vi "sub2.vi"(10 "regular expression":string, 11 "Array":T1(array[cluster])) -> (3 "Tunnel out":refnum<vi>)   [LabVIEW 2020, in "CSM-Helper.lvclass"]
uses:
  CSM-Helper.lvclass
  a22f351f-3913-4f37-956c-d0ef2cfe06c6.vi
  cf7c94ff-430a-4fdd-9615-a1dbd9b9f88c.vi
  a22f351f-3913-4f37-956c-d0ef2cfe06c6.vi/eb2405bd-5b2e-436b-9bb3-692ecf4a9268.vi
  a22f351f-3913-4f37-956c-d0ef2cfe06c6.vi/c8ad12e3-5e6d-40e1-92e0-1426ef45ec41.vi
  a22f351f-3913-4f37-956c-d0ef2cfe06c6.vi/effcbc1a-e97c-42d4-b61f-d821de102707.vi
  cf7c94ff-430a-4fdd-9615-a1dbd9b9f88c.vi/eb2405bd-5b2e-436b-9bb3-692ecf4a9268.vi
  cf7c94ff-430a-4fdd-9615-a1dbd9b9f88c.vi/c8ad12e3-5e6d-40e1-92e0-1426ef45ec41.vi
  cf7c94ff-430a-4fdd-9615-a1dbd9b9f88c.vi/effcbc1a-e97c-42d4-b61f-d821de102707.vi
  CSM-Helper.lvclass/CSM-Helper.ctl
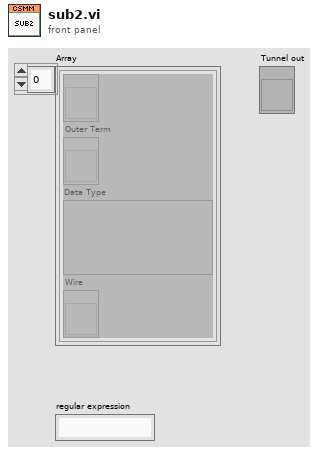
[diagram p1: front panel]
types:
  T1 = cluster{refnum<vi>, "Outer Term":refnum<vi>, "Data Type":variant, "Wire":refnum<vi>}[]
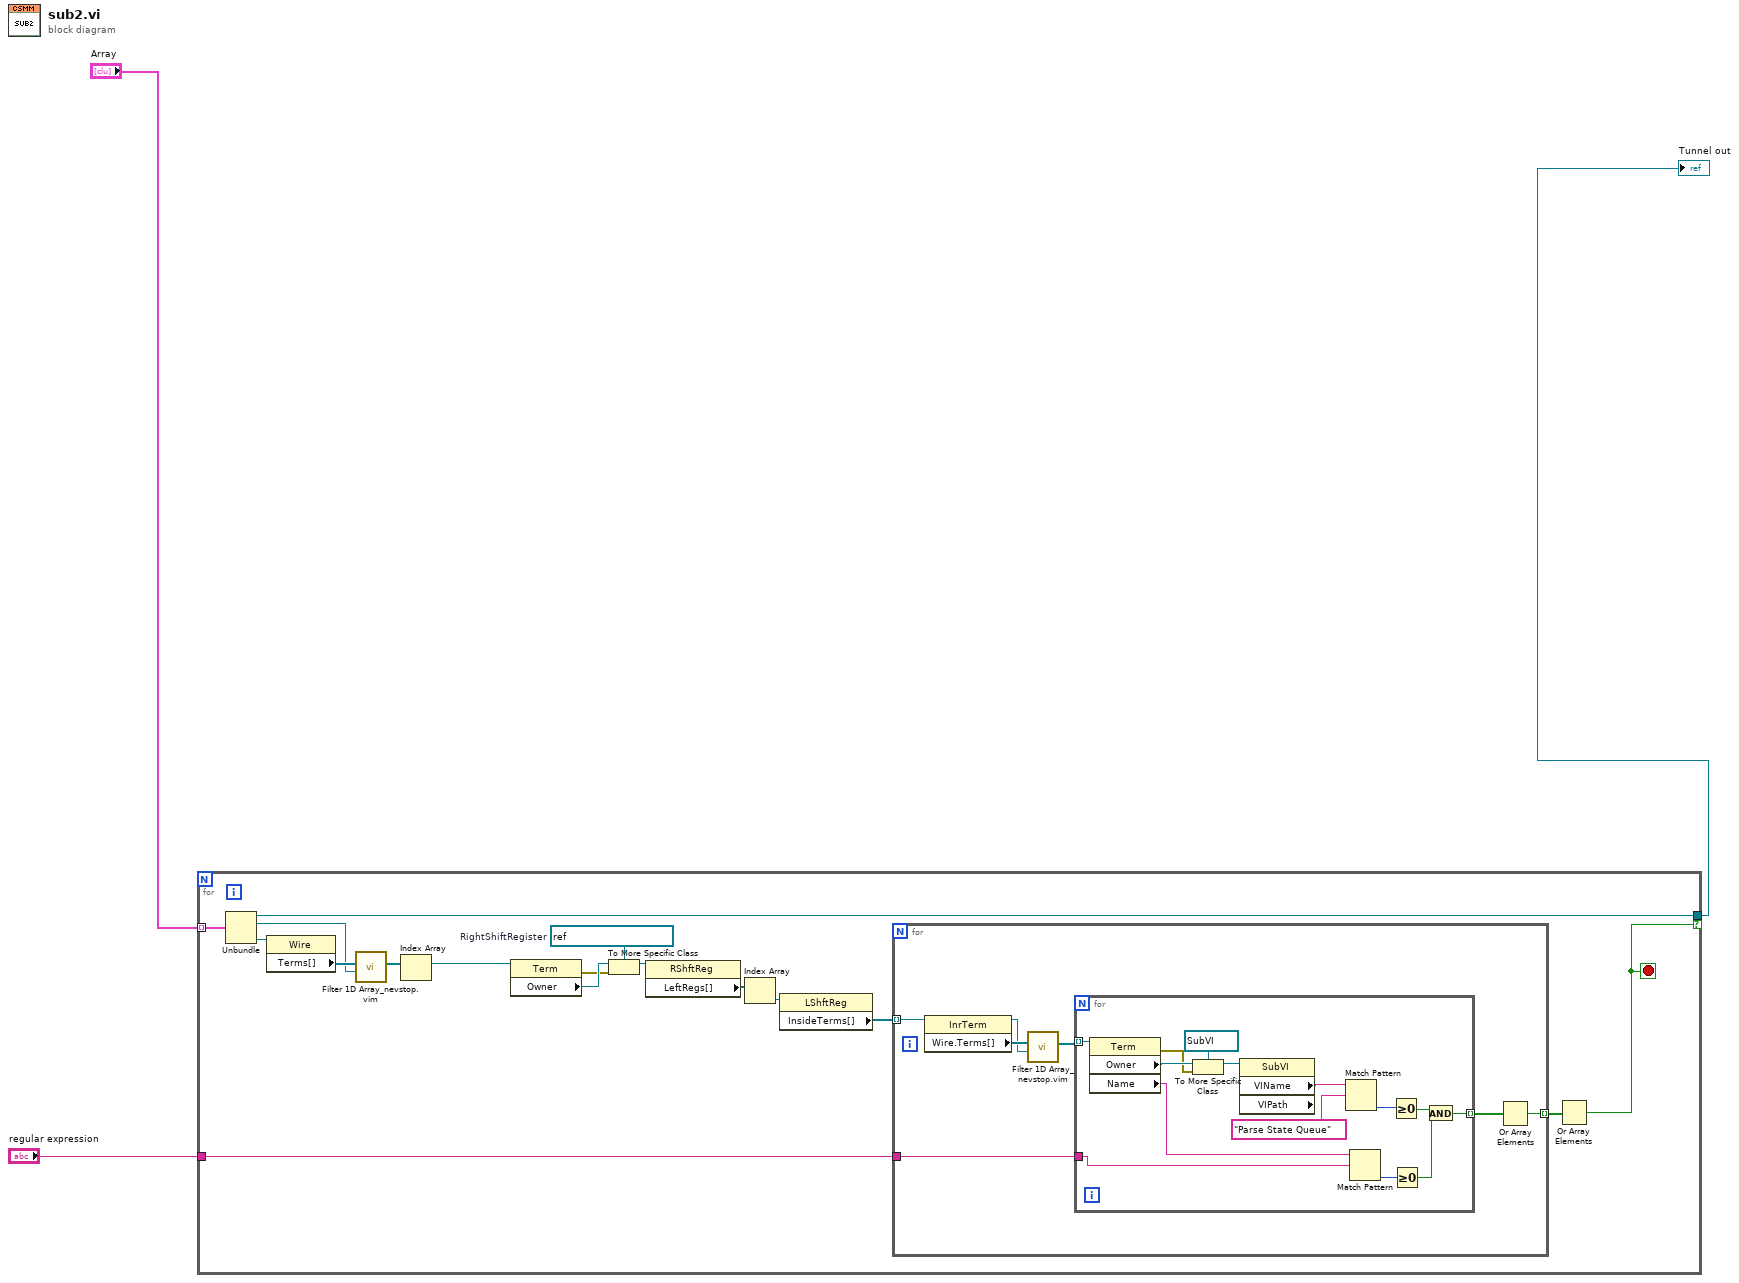
[diagram p0: block diagram]
diagram:
  n1 = for {
    tunnel: "Array" -> [w20] mode=indexing
    tunnel: [w19] -> w3 if=w7
    tunnel: "regular expression" -> [w6]
    stop <- w7 stop-if-true
    w13 = refnum<vi> refnum  # RightShiftRegister
    n2 = Unbundle(w20) -> (w19:refnum<vi>, "Outer Term"=w16:refnum<vi>, "Wire"=w17:refnum<vi>)  [unwired: 1 out]
    n3 = property class="Wire"(reference=w17) -> ("Terms[]"=w18:refnum<vi>[])  [unwired: 1 in, 2 out]
    n4 = call "Filter 1D Array_nevstop.vim"("items to filter"=w16, "array"=w18) -> ("filtered array"=w15:refnum<vi>[])  [unwired: 4 in, 1 out]
    n5 = Index Array(array=w15) -> (element=w14:refnum<vi>)  [unwired: 1 in]
    n6 = property class="Term"(reference=w14) -> (error out=w4:errorcluster, "Owner"=w5:refnum<vi>)  [unwired: 1 in, 1 out]
    n7 = To More Specific Class(target class=w13, reference=w5, error in=w4) -> (specific class reference=w12:refnum<vi>)  [unwired: 1 out]
    n8 = property class="RShftReg"(reference=w12) -> ("LeftRegs[]"=w11:refnum<vi>[])  [unwired: 1 in, 2 out]
    n9 = Index Array(array=w11) -> (element=w10:refnum<vi>)  [unwired: 1 in]
    n10 = property class="LShftReg"(reference=w10) -> ("InsideTerms[]"=w9:refnum<vi>[])  [unwired: 1 in, 2 out]
    n11 = for {
      tunnel: w9 -> [w27] mode=indexing
      tunnel: [w22] -> w8 mode=indexing
      tunnel: w6 -> [w21]
      n12 = property class="InrTerm"(reference=w27) -> (reference out=w25:refnum<vi>, "Wire.Terms[]"=w26:refnum<vi>[])  [unwired: 1 in, 1 out]
      n13 = call "Filter 1D Array_nevstop.vim"("items to filter"=w25, "array"=w26) -> ("filtered array"=w24:refnum<vi>[])  [unwired: 4 in, 1 out]
      n14 = for {
        tunnel: [w30] -> w23 mode=indexing
        tunnel: w24 -> [w29] mode=indexing
        tunnel: w21 -> [w28]
        n15 = property class="Term"(reference=w29) -> (error out=w39:errorcluster, "Owner"=w41:refnum<vi>, "Name"=w35:string)  [unwired: 1 in, 1 out]
        n16 = To More Specific Class(target class=refnum<vi> refnum ("Parse State Queue"), reference=w41, error in=w39) -> (specific class reference=w38:refnum<vi>)  [unwired: 1 out]
        n17 = property class="SubVI" props=["VIName", "VIPath"](reference=w38) -> ("VIName"=w37:string)  [unwired: 1 in, 3 out]
        n18 = Match Pattern(string=w37, regular expression="Parse State Queue") -> (offset past match=w34:i32)  [unwired: 1 in, 3 out]
        n19 = Match Pattern(string=w35, regular expression=w28) -> (offset past match=w33:i32)  [unwired: 1 in, 3 out]
        n20 = Greater Or Equal To 0?(x=w34) -> (x >= 0?=w32:bool)
        n21 = Greater Or Equal To 0?(x=w33) -> (x >= 0?=w31:bool)
        n22 = And(x=w32, y=w31) -> (x .and. y?=w30:bool)
      }
      n23 = Or Array Elements(Boolean array=w23) -> (logical OR=w22:bool)
    }
    n24 = Or Array Elements(Boolean array=w8) -> (logical OR=w7:bool)
  }
  "Tunnel out" <- w3
